vi "movemotor.vi"(8 "error in (no error)":errorcluster, 10 "motor voltage":dbl, 11 "simulated in":refnum<class "simulated.lvclass">) -> (0 "error out":errorcluster, 3 "simulated out":refnum<class "simulated.lvclass">)   [LabVIEW 2015, in "simulated.lvclass"]
uses:
  simulated.lvclass
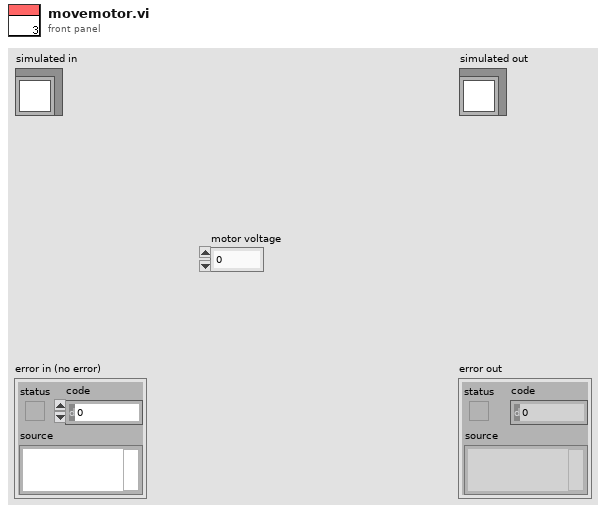
[diagram p1: front panel]
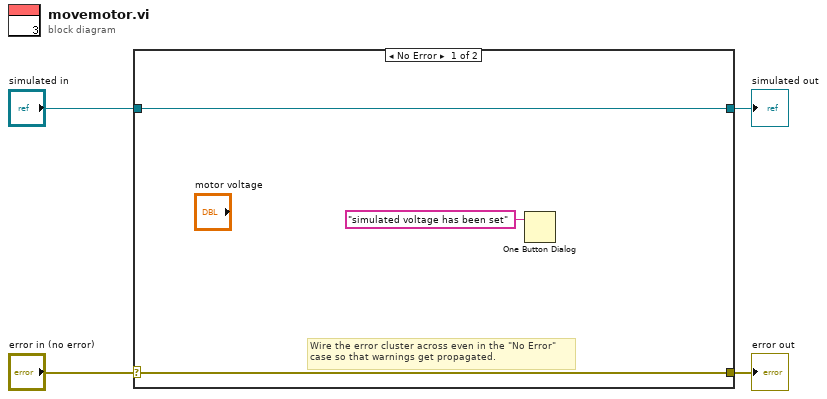
[diagram p0: block diagram]
diagram:
  n1 = case shown="No Error" "error in (no error)" {
    selector: "error in (no error)" -> [w6 w9]
    tunnel: [w6 w9] -> w3
    tunnel: [w7 w8] -> w1
    tunnel: "simulated in" -> [w7 w8]
    frame No Error {
      # "Wire the error cluster across even in the \"No Error\"\ncase so that warnings get propagated."
      n2 = One Button Dialog(message="simulated voltage has been set") -> ()  [unwired: 1 in, 1 out]
    }
    frame Error {
    }
  }
  "error out" <- w3
  "simulated out" <- w1
